vi "GetProjectorParameters.vi"(5 "error in (no error)":errorcluster, 6 "Camera Reference in":refnum<k24>) -> (0 "PowerLevel (High Normal Low)":u8(ring) items=["High", "Normal", "Low"], 1 "FringeCodingMode (Fast Accurate Translucent Reflective)":u8(ring) items=["Fast", "Accurate", "Translucent", "Reflective"], 2 "error out":errorcluster, 3 "Camera Reference out":refnum<k24>, 4 "AntiFlickerMode (Off AC50Hz AC60Hz)":u8(ring) items=["Off", "AC50Hz", "AC60Hz"])   [LabVIEW 2023]
uses:
  C:/Mech-Mind/Mech-Eye SDK-2.5.0-b5-dev-01-03/API/dll/net48/MechEyeApiNet.dll
  dll/net48/MechEyeApiNet.dll
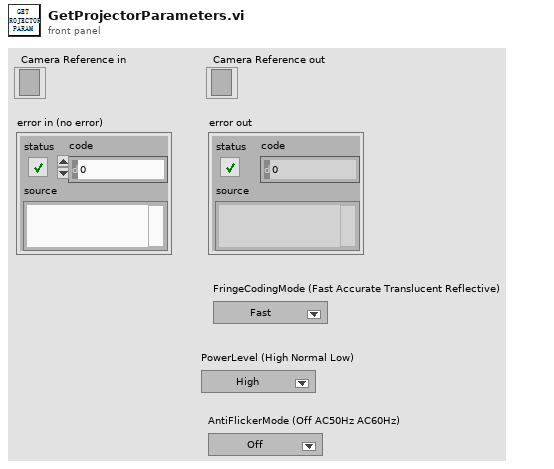
[diagram p1: front panel]
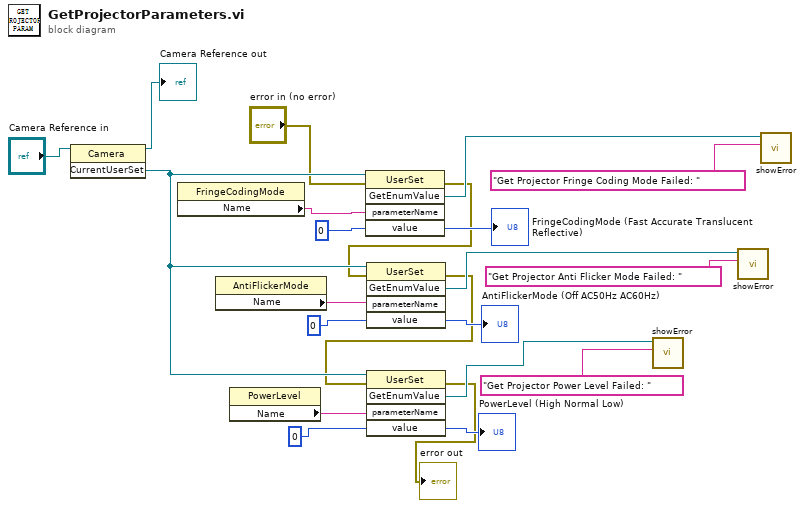
[diagram p0: block diagram]
diagram:
  n1 = invoke class="Camera" method="CurrentUserSet"(reference="Camera Reference in") -> (reference out=→"Camera Reference out":refnum<k24>, "CurrentUserSet"=w11:refnum<k24>)  [unwired: 2 in, 1 out]
  n2 = property class="FringeCodingMode"() -> ("Name"=w19:string)  [unwired: 2 in, 2 out]
  n3 = property class="AntiFlickerMode"() -> ("Name"=w15:string)  [unwired: 2 in, 2 out]
  n4 = property class="PowerLevel"() -> ("Name"=w10:string)  [unwired: 2 in, 2 out]
  n5 = invoke class="UserSet" method="GetEnumValue"(reference=w11, error in="error in (no error)", "parameterName"=w19, "value"=0) -> (error out=w5:errorcluster, "GetEnumValue"=w16:refnum<k24>, "value"=→"FringeCodingMode (Fast Accurate Translucent Reflective)":i32)  [unwired: 1 in, 2 out]
  n6 = invoke class="UserSet" method="GetEnumValue"(reference=w11, error in=w5, "parameterName"=w15, "value"=0) -> (error out=w4:errorcluster, "GetEnumValue"=w13:refnum<k24>, "value"=→"AntiFlickerMode (Off AC50Hz AC60Hz)":i32)  [unwired: 1 in, 2 out]
  n7 = invoke class="UserSet" method="GetEnumValue"(reference=w11, error in=w4, "parameterName"=w10, "value"=0) -> (error out=→"error out":errorcluster, "GetEnumValue"=w7:refnum<k24>, "value"=→"PowerLevel (High Normal Low)":i32)  [unwired: 1 in, 2 out]
  n8 = call "showError.vi"("String"="Get Projector Power Level Failed: ", "MMind.Eye.ErrorStatus"=w7) -> ()  [unwired: 10 in]
  n9 = call "showError.vi"("String"="Get Projector Anti Flicker Mode Failed: ", "MMind.Eye.ErrorStatus"=w13) -> ()  [unwired: 10 in]
  n10 = call "showError.vi"("String"="Get Projector Fringe Coding Mode Failed: ", "MMind.Eye.ErrorStatus"=w16) -> ()  [unwired: 10 in]
